vi "Erf_KnifeEdgeFitting.vi"(3 "output control":T1, 4 "data":T2, 5 "X":dbl[](array[numeric]), 6 "a":dbl[](array[numeric])) -> (0 "error out":errorcluster, 1 "f'(X,a)":dbl[][](array[numeric]), 2 "f(X,a)":dbl[](array[numeric]))   [LabVIEW 2011]
doc: "This template is the starting point for creating a model function to be passed to the Nonlinear Curve Fit.vi."
uses:
  <vilib>/gmath/NumericalOptimization/objective function data.ctl
  <vilib>/gmath/NumericalOptimization/LM_output select.ctl
  <vilib>/gmath/NI_Gmath.lvlib
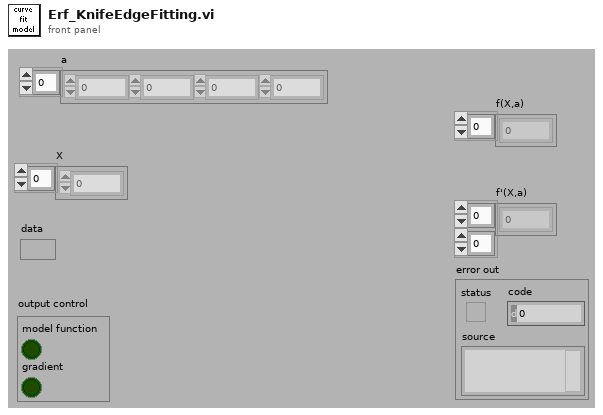
[diagram p1: front panel]
types:
  T1 = typedef "NI_Gmath.lvlib/LM_output select.ctl" = cluster{"model function":bool, "gradient":bool}
  T2 = typedef "NI_Gmath.lvlib/objective function data.ctl" = variant
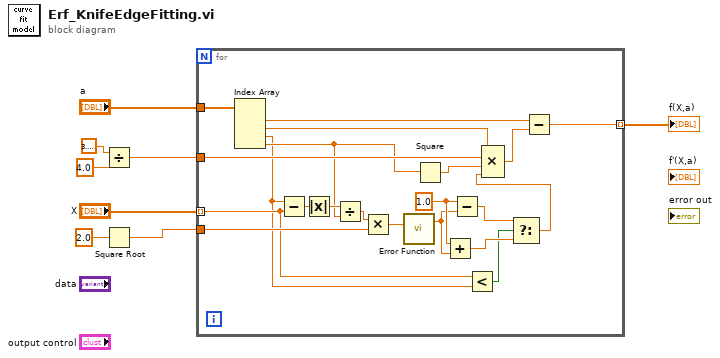
[diagram p0: block diagram]
diagram:
  n1 = Divide(x=3.141592653589793, y=4.0) -> (x/y=w1:dbl)
  n2 = Square Root(x=2.0) -> (sqrt(x)=w5:dbl)
  n3 = for {
    tunnel: "a" -> [w29]
    tunnel: "X" -> [w11] mode=indexing
    tunnel: w5 -> [w17]
    tunnel: [w25] -> w4 mode=indexing
    tunnel: w1 -> [w24]
    w16 = 1.0 ("x")
    n4 = Index Array(array=w29) -> (element #1=w28:dbl, element #2=w26:dbl, element #3=w10:dbl, element #4=w19:dbl)  [unwired: 4 in]
    n5 = Subtract(x=w10, y=w11) -> (x-y=w22:dbl)
    n6 = Absolute Value(x=w22) -> (abs(x)=w21:dbl)
    n7 = Divide(x=w21, y=w19) -> (x/y=w20:dbl)
    n8 = Multiply(x=w20, y=w17) -> (x*y=w18:dbl)
    n9 = call <vilib>:"Error Function.vi"("x"=w18) -> ("erf(x)"=w15:dbl)  [unwired: 2 in]
    n10 = Square(x=w19) -> (x^2=w23:dbl)
    n11 = Add(x=w16, y=w15) -> (x+y=w13:dbl)
    n12 = Subtract(x=w16, y=w15) -> (x-y=w14:dbl)
    n13 = Less?(x=w11, y=w10) -> (x < y?=w12:bool)
    n14 = Select(t=w14, s=w12, f=w13) -> (s? t:f=w9:dbl)
    n15 = Compound Arithmetic op=MULTIPLY(w26, w24, w23, w9) -> (w27:dbl)
    n16 = Subtract(x=w28, y=w27) -> (x-y=w25:dbl)
  }
  "f(X,a)" <- w4
